vi "Actor Core.vi"(8 "error in":errorcluster, 11 "Launch IMAQ Display in":refnum<class "HIJ Single Cam App Demo.lvclass">) -> (0 "error out":errorcluster, 3 "Actor out":refnum<class "Actor.lvclass">)   [LabVIEW 2014, in "HIJ Single Cam App Demo.lvlib" / "HIJ Single Cam App Demo.lvclass"]
doc: "(<B>Filename</B>: Actor Framework.lvlib:Actor.lvclass:Actor Core.vi)\n\nReceives messages to the actor, reacts to them, and initiates any error handling that may shut the actor down.\n\nDescendant classes may override this VI to append parallel tasks for the actor to complete while it handles messages. Overrides use the Call Parent Method node."
uses:
  HIJ Single Cam App Demo.lvclass
  <vilib>/ActorFramework/Actor/Actor.lvclass
  Display Actors/HIJ IMAQdx Display/AF IMAQ Display/HIJ IMAQdx Display.lvclass
  Analyze/Analyze Classes/Analyze Diviation/Analyze BeamDeviation.lvclass
  Analyze/Results and Overlays/Results Beam Deviation/Analyze Results Beam Deviation.lvclass
  Analyze/Analyze Classes/Analyze Distanz/Analyze Distanz.lvclass
  Analyze/Results and Overlays/Results Distance/Analyze Results Distanz.lvclass
  Camera Actors/IMAQdx Actor/IMAQdx Actor/IMAQdx Actor.lvclass
  Analyze/Analyze Classes/Analyze Fluence/Analyze Fluence.lvclass
  Analyze/Results and Overlays/Results Fluence/Analyze Results Fluence.lvclass
  Analyze/Analyze Parameter/Analyze Parameter Energy/Analyze Parameter Energy.lvclass
  Analyze/Analyze Parameter/Analyze Parameter Fluence/Analyze Parameter Fluence.lvclass
  Display Actors/HIJ Vision Display/HIJ Vision Display/HIJ Vision Display.lvclass/HIJ Vision Display.ctl
  Analyze/Analyze Parameter/Analyze Parameter Energy/Analyze Parameter Energy.lvclass/Analyze Parameter Energy.ctl
  HIJ Single Cam App Demo.lvclass/HIJ Single Cam App Demo.ctl
  Analyze/Results and Overlays/Results Fluence/Analyze Results Fluence.lvclass/Analyze Results Fluence.ctl
  HIJ Vision Application/HIJ Vision Application/HIJ Vision Application.lvclass/HIJ Vision Application.ctl
  HIJ Vision Camera App/HIJ Vision Camera App/HIJ Vision Camera App.lvclass/HIJ Vision Camera App.ctl
  Shared Code/Viewable Actor/ViewableActor/ViewableActor.lvclass/ViewableActor.ctl
  <vilib>/ActorFramework/Actor/Actor.lvclass/Actor.ctl
  <vilib>/ActorFramework/Message Enqueuer/Message Enqueuer.lvclass/Message Enqueuer.ctl
  HIJ Vision Camera App/HIJ Vision Camera App Messages/Menu Selection Msg/Menu Selection Msg.lvclass/Menu Selection Msg.ctl
  HIJ Vision Application/HIJ Vision Application Messages/Set Parameter Msg/Set Parameter Msg.lvclass/Set Parameter Msg.ctl
  Analyze/Analyze Parameter/Analyze Parameter Energy/Write Energy.vi
  Analyze/Results and Overlays/Results Fluence/Write UI Ref Max F.vi
  Display Actors/HIJ Vision Display/HIJ Vision Display/Write Save Report_.vi
  HIJ Vision Application/HIJ Vision Application/Write SubPnl for Display.vi
  HIJ Vision Camera App/HIJ Vision Camera App/Write Child Menu.vi
  HIJ Vision Application/HIJ Vision Application/Write HIJ Vision Display.vi
  HIJ Vision Application/HIJ Vision Application/Write Analyze Objs.vi
  HIJ Vision Camera App/HIJ Vision Camera App/Write Camera Actor.vi
  Shared Code/Viewable Actor/ViewableActor/Write UI VI Ref.vi
  HIJ Vision Camera App/HIJ Vision Camera App/Write SubPnl for Settings.vi
  <vilib>/ActorFramework/Message Enqueuer/Init from Existing Queue.vi
  <vilib>/ActorFramework/Message Enqueuer/Enqueue.vi
  <vilib>/ActorFramework/Message Priority Queue/Priority Enqueue.vi
  <vilib>/ActorFramework/Message Enqueuer/Message Enqueuer.lvclass
  HIJ Vision Camera App/HIJ Vision Camera App Messages/Menu Selection Msg/Menu Selection Msg.lvclass
  HIJ Vision Application/HIJ Vision Application Messages/Set Parameter Msg/Set Parameter Msg.lvclass
  <vilib>/ActorFramework/Stop Msg/Stop Msg.lvclass
  HIJ Vision Camera App/HIJ Vision Camera App/HIJ Vision Camera App.lvclass
panel:
  in  "Stop Button":bool
  in  "@Energy":dbl[unit]=10.0
  out "Max Fluence":dbl[unit] format="%#_3g"
  # "HIER wird Settings Dialog \nerscheinen, wenn Du die \nReferenz dieses Panels\nim \"Actor Core.vi\"\nan die Klassen Property\n \"SubPnl for Settings\"\nübergibst."
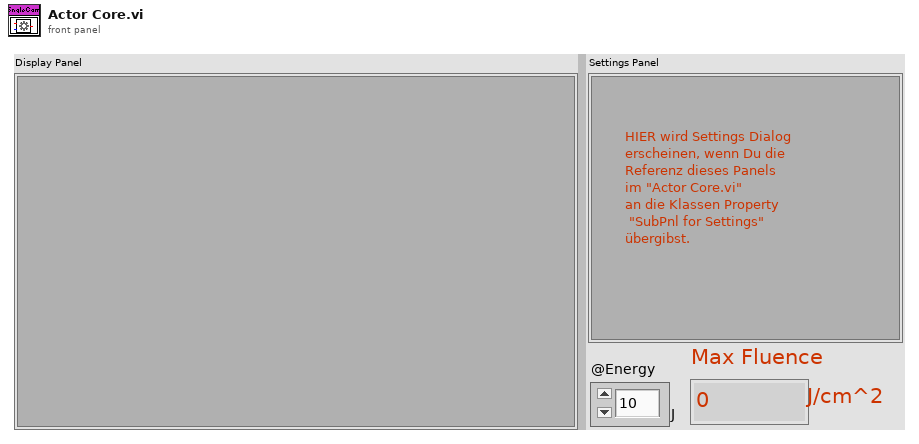
[diagram p1: front panel]
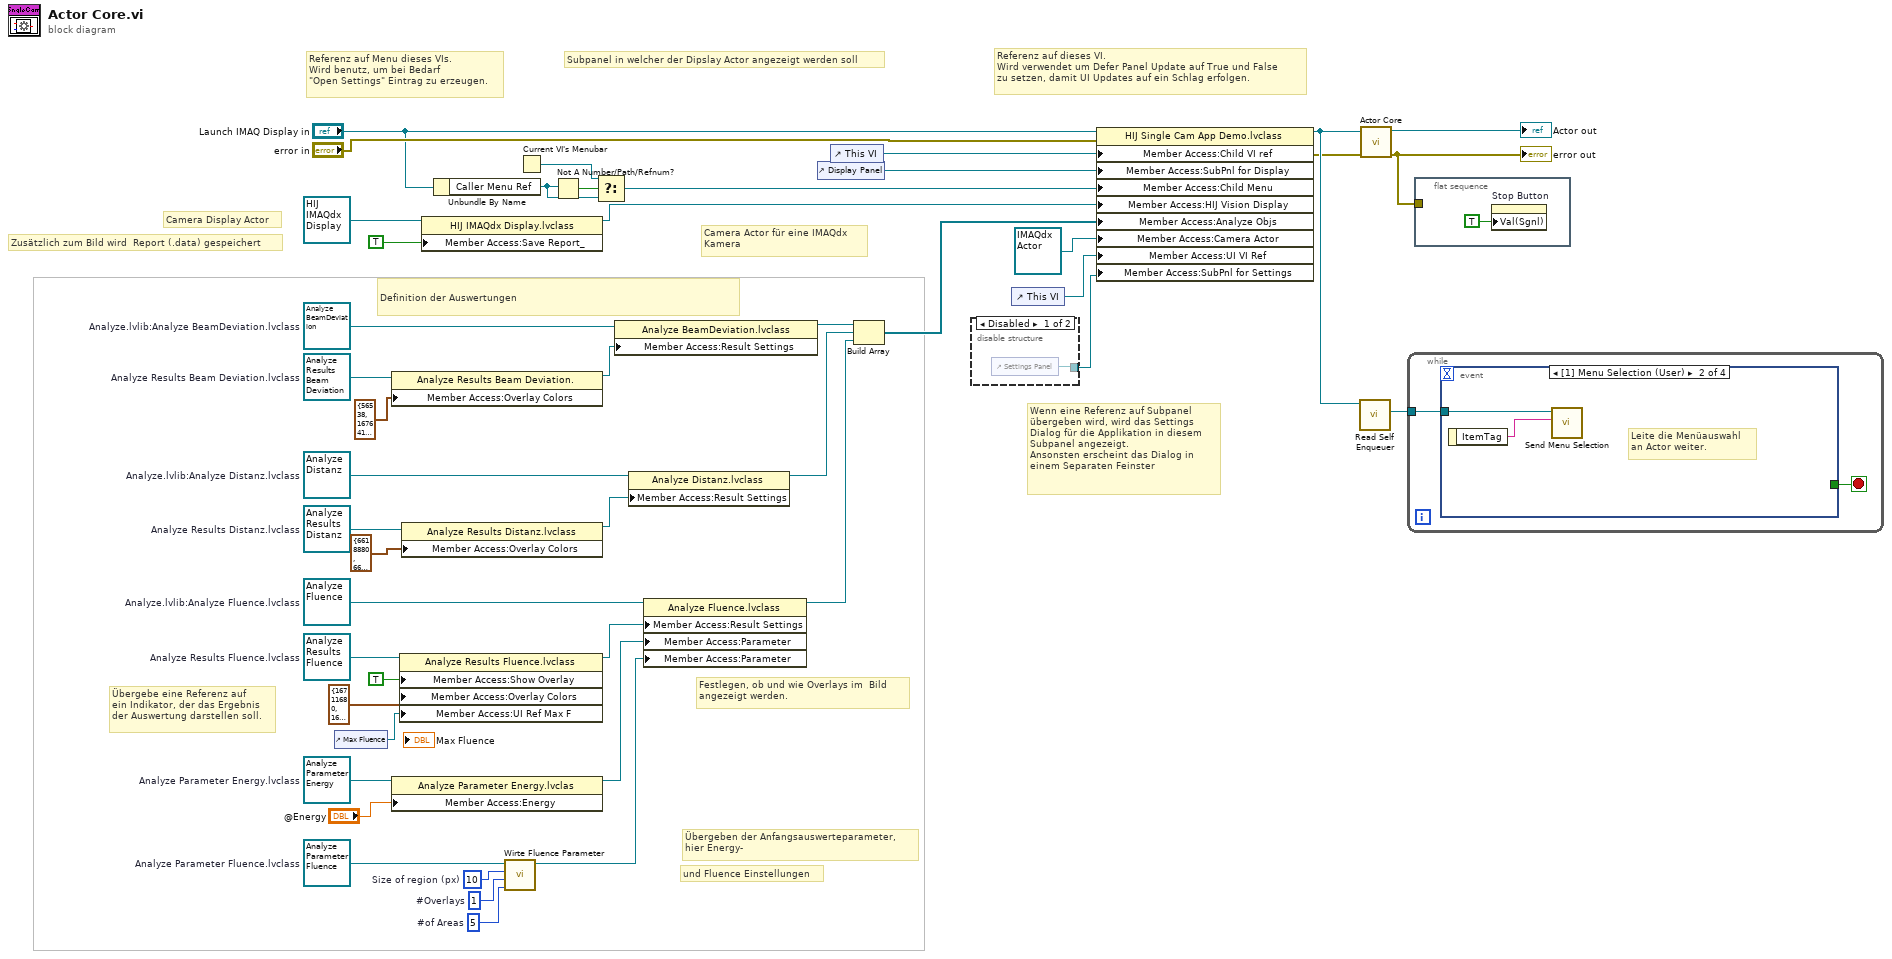
[diagram p0: block diagram]
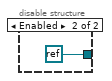
[diagram p2: hidden frame]
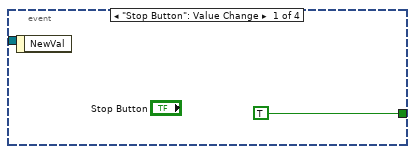
[diagram p3: hidden frame]
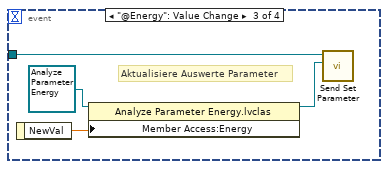
[diagram p4: hidden frame]
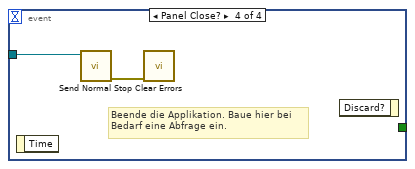
[diagram p5: hidden frame]
diagram:
  w10 = 10  # Size of region (px)
  w11 = 1  # #Overlays
  w12 = 5  # #of Areas
  w14 = refnum<class "Analyze Parameter Fluence.lvclass"> refnum  # Analyze Parameter Fluence.lvclass
  w17 = refnum<class "Analyze Parameter Energy.lvclass"> refnum  # Analyze Parameter Energy.lvclass
  w25 = refnum<class "Analyze Results Fluence.lvclass"> refnum  # Analyze Results Fluence.lvclass
  w26 = refnum<class "Analyze Fluence.lvclass"> refnum  # Analyze.lvlib:Analyze Fluence.lvclass
  w36 = refnum<class "Analyze Results Distanz.lvclass"> refnum  # Analyze Results Distanz.lvclass
  w37 = refnum<class "Analyze Distanz.lvclass"> refnum  # Analyze.lvlib:Analyze Distanz.lvclass
  w39 = refnum<class "Analyze Results Beam Deviation.lvclass"> refnum  # Analyze Results Beam Deviation.lvclass
  w40 = refnum<class "Analyze BeamDeviation.lvclass"> refnum  # Analyze.lvlib:Analyze BeamDeviation.lvclass
  # "Wenn eine Referenz auf Subpanel\nübergeben wird, wird das Settings\nDialog für die Applikation in diesem\nSubpanel angezeigt.\nAnsonsten erscheint das Dialog in \neinem Separaten Feinster"
  # "Camera Actor für eine IMAQdx\nKamera"
  # "Referenz auf Menu dieses VIs.\nWird benutz, um bei Bedarf \n\"Open Settings\" Eintrag zu erzeugen."
  # "Übergebe eine Referenz auf\nein Indikator, der das Ergebnis\nder Auswertung darstellen soll."
  # "und Fluence Einstellungen"
  # "Übergeben der Anfangsauswerteparameter, \nhier Energy-"
  # "Festlegen, ob und wie Overlays im  Bild \nangezeigt werden."
  # "Referenz auf dieses VI.\nWird verwendet um Defer Panel Update auf True und False\nzu setzen, damit UI Updates auf ein Schlag erfolgen."
  # "Definition der Auswertungen"
  # "Camera Display Actor"
  # "Zusätzlich zum Bild wird  Report (.data) gespeichert"
  # "Subpanel in welcher der Dipslay Actor angezeigt werden soll"
  n1 = control-ref of="Max Fluence"() -> (w22:refnum<vi>)
  n2 = property class="Analyze Results Beam Deviation."(reference=w39, "Member Access:Overlay Colors"=cluster{"Border":u32, "Text":u32} {"Border"=56538, "Text"=16764160} ("Colors")) -> (reference out=w19:refnum<class "Analyze Results Beam Deviation.lvclass">)  [unwired: 1 in, 1 out]
  n3 = property class="Analyze Parameter Energy.lvclas"(reference=w17, "Member Access:Energy"="@Energy") -> (reference out=w15:refnum<class "Analyze Parameter Energy.lvclass">)  [unwired: 1 in, 1 out]
  n4 = property class="Analyze Results Fluence.lvclass"(reference=w25, "Member Access:Show Overlay"=TRUE ("bOverlay"), "Member Access:Overlay Colors"=cluster{"Border":u32, "Text":u32} {"Border"=16711680, "Text"=16448250} ("Colors"), "Member Access:UI Ref Max F"=w22) -> (reference out=w21:refnum<class "Analyze Results Fluence.lvclass">)  [unwired: 1 in, 1 out]
  n5 = property class="Analyze Results Distanz.lvclass"(reference=w36, "Member Access:Overlay Colors"=cluster{"Border":u32, "Text":u32} {"Border"=6618880, "Text"=6618880} ("Colors")) -> (reference out=w18:refnum<class "Analyze Results Distanz.lvclass">)  [unwired: 1 in, 1 out]
  n6 = property class="HIJ IMAQdx Display.lvclass"(reference=refnum<class "HIJ IMAQdx Display.lvclass"> refnum ("IMAQ Display.lvlib:IMAQ Display.lvclass"), "Member Access:Save Report_"=TRUE ("Save Report_")) -> (reference out=w27:refnum<class "HIJ IMAQdx Display.lvclass">)  [unwired: 1 in, 1 out]
  n7 = Unbundle By Name("Launch IMAQ Display in") -> ("Caller Menu Ref"=w1:refnum<k9>)
  n8 = call "Wirte Fluence Parameter.vi"("#of Areas"=w12, "#Overlays"=w11, "Size of region (px)"=w10, "Analyze Parameter Fluence in"=w14) -> ("Analyze Parameter Fluence out"=w13:refnum<class "Analyze Parameter Fluence.lvclass">)  [unwired: 7 in]
  n9 = Current VI's Menubar() -> (w2:refnum<k9>)
  n10 = Not A Number/Path/Refnum?(number/path/refnum=w1) -> (NaN/Path/Refnum?=w4:bool)
  n11 = Select(t=w2, s=w4, f=w1) -> (s? t:f=w3:refnum<k9>)
  n12 = property class="Analyze BeamDeviation.lvclass"(reference=w40, "Member Access:Result Settings"=w19) -> (reference out=w20:refnum<class "Analyze BeamDeviation.lvclass">)  [unwired: 1 in, 1 out]
  n13 = property class="Analyze Distanz.lvclass"(reference=w37, "Member Access:Result Settings"=w18) -> (reference out=w9:refnum<class "Analyze Distanz.lvclass">)  [unwired: 1 in, 1 out]
  n14 = property class="Analyze Fluence.lvclass"(reference=w26, "Member Access:Result Settings"=w21, "Member Access:Parameter"=w15, "Member Access:Parameter"=w13) -> (reference out=w8:refnum<class "Analyze Fluence.lvclass">)  [unwired: 1 in, 1 out]
  n15 = control-ref of="Display Panel"() -> (w29:refnum<vi>)
  n16 = control-ref of="This VI"() -> (w33:refnum<vi>)
  n17 = Build Array(w20, w9, w8) -> (w30:refnum<class "Analyze BaseClass.lvclass">[])
  n18 = disable-structure shown="Disabled" {
    disable-tunnel: [w46 refnum<k0> refnum] -> w7
    frame Disabled {
      n19 = control-ref of="Settings Panel"() -> (w46:refnum<vi>)
    }
    frame Enabled {
    }
  }
  n20 = control-ref of="This VI"() -> (w6:refnum<vi>)
  n21 = property class="HIJ Single Cam App Demo.lvclass"(reference="Launch IMAQ Display in", error in="error in", "Member Access:Child VI ref"=w33, "Member Access:SubPnl for Display"=w29, "Member Access:Child Menu"=w3, "Member Access:HIJ Vision Display"=w27, "Member Access:Analyze Objs"=w30, "Member Access:Camera Actor"=refnum<class "IMAQdx Actor.lvclass"> refnum ("IMAQdx Actor.lvlib:IMAQdx Actor.lvclass"), "Member Access:UI VI Ref"=w6, "Member Access:SubPnl for Settings"=w7) -> (reference out=w34:refnum<class "HIJ Single Cam App Demo.lvclass">, error out=w31:errorcluster)
  n22 = call <vilib>:"Read Self Enqueuer.vi"("Actor"=w34) -> ("Self Enqueuer"=w42:refnum<class "Message Enqueuer.lvclass">)  [unwired: 10 in]
  n23 = call-parent "Actor Core.vi"("error in"=w31, "HIJ Vision Camera App In"=w34) -> ("error out"=w43:errorcluster, "Actor out"=→"Actor out":refnum<class "Actor.lvclass">)  [unwired: 8 in]
  "error out" <- w43
  n24 = while {
    tunnel: w42 -> [w48]
    stop <- w49 stop-if-true
    n25 = event shown="[1] Menu Selection (User)" {
      selector: _ -> [_ _ _ _]
      dyn-events: _ -> [_ _ _ _]
      timeout: _ -> [_ _ _ _]
      tunnel: [TRUE _ _ _] -> w49
      tunnel: w48 -> [_ w51 w54 w58]
      event "Stop Button": Value Change {
        n26 = event-data() -> ()  [unwired: 1 in, 1 out]
      }
      event Menu Selection (User) {
        # "Leite die Menüauswahl \nan Actor weiter."
        n27 = event-data() -> ("ItemTag"=w52:string)  [unwired: 1 in]
        n28 = call "Send Menu Selection.vi"("MenuTag"=w52, "Message Enqueuer"=w51) -> ()  [unwired: 8 in, 2 out]
      }
      event "@Energy": Value Change {
        # "Aktualisiere Auswerte Parameter"
        n29 = event-data() -> ("NewVal"=w55:dbl[unit])  [unwired: 1 in]
        n30 = property class="Analyze Parameter Energy.lvclas"(reference=refnum<class "Analyze Parameter Energy.lvclass"> refnum ("Analyze Parameter Energy.lvclass"), "Member Access:Energy"=w55) -> (reference out=w53:refnum<class "Analyze Parameter Energy.lvclass">)  [unwired: 1 in, 1 out]
        n31 = call "Send Set Parameter.vi"("Parameter"=w53, "Message Enqueuer"=w54) -> ()  [unwired: 8 in, 2 out]
      }
      event Panel Close? {
        # "Beende die Applikation. Baue hier bei\nBedarf eine Abfrage ein."
        n32 = event-data() -> ()  [unwired: 1 in, 1 out]
        n33 = call <vilib>:"Send Normal Stop.vi"("Message Enqueuer"=w58) -> ("error out"=w57:errorcluster)  [unwired: 10 in]
        n34 = call <vilib>:"Clear Errors.vi"("error in (no error)"=w57) -> ()  [unwired: 5 in, 2 out]
        n35 = event-data() -> ()  [unwired: 2 in, 1 out]
      }
    }
  }
  n36 = flat-sequence {
    tunnel: w43 -> [_]
    frame #0 {
      n37 = property on="Stop Button" class="Bool (strict)"("Val(Sgnl)"=TRUE) -> ()  [unwired: 2 in, 2 out]
    }
  }
